vi "PAM Unix to LabVIEW Time.vi"(11 "Unix":dbl=1440541207.603 format="%#_13g") -> (3 "Labview Timestamp":timestamp)   [LabVIEW 2020]
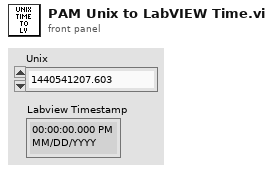
[diagram p1: front panel]
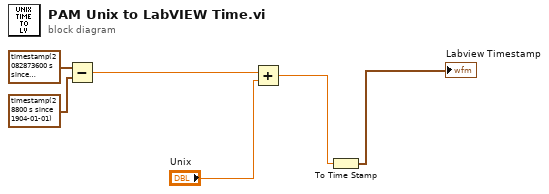
[diagram p0: block diagram]
diagram:
  n1 = Subtract(x=timestamp(2082873600 s since 1904-01-01), y=timestamp(28800 s since 1904-01-01)) -> (x-y=w3:dbl)
  n2 = Add(x=w3, y="Unix") -> (x+y=w2:dbl)
  n3 = To Time Stamp(1:w2) -> (0:→"Labview Timestamp":timestamp)
